vi "From JSON.vi"(8 "error in (no error)":errorcluster, 10 "<JSON>Config>":string, 11 "Configuration Base in":refnum<class "Config Base.lvclass">) -> (0 "error out":errorcluster, 3 "Configuration Base out":refnum<class "Config Base.lvclass">)   [LabVIEW 2023, in "HAL GOOP4.lvlib" / "Config Base.lvclass"]
uses:
  Config Base.lvclass
  Config Base.lvclass/Config Base.ctl
  <vilib>/ErrorRing/Error Ring.xnode
  <vilib>/Utility/error.llb/Error Cluster From Error Code.vi
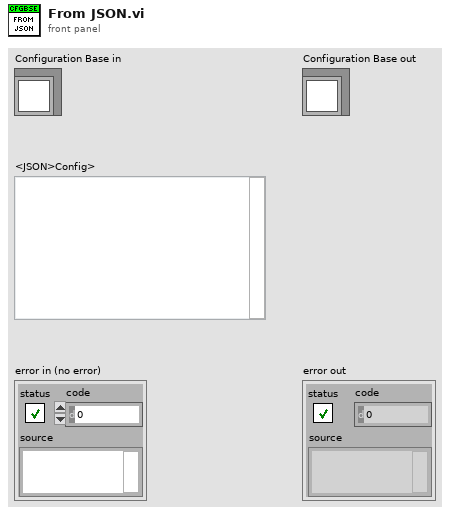
[diagram p1: front panel]
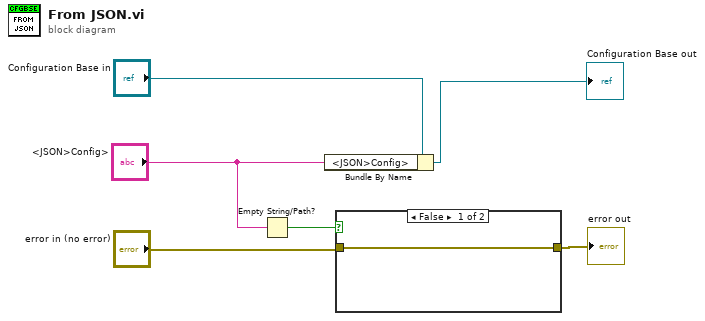
[diagram p0: block diagram]
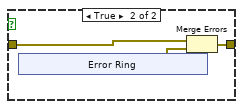
[diagram p2: hidden frame]
diagram:
  n1 = Empty String/Path?(string/path="<JSON>Config>") -> (empty?=w1:bool)
  n2 = Bundle By Name(cluster="Configuration Base in", "<JSON>Config>"="<JSON>Config>") -> (→"Configuration Base out":refnum<class "Config Base.lvclass">)
  n3 = case shown="False" w1 {
    tunnel: "error in (no error)" -> [w7 w8]
    tunnel: [w7 w10] -> w3
    frame False {
    }
    frame True {
      n4 = xnode "Error Ring"() -> ("error out"=w9:errorcluster)
      n5 = Merge Errors(w8, w9) -> (w10:errorcluster)
    }
  }
  "error out" <- w3
